vi "Read BMP File Data (excel).vi"(8 "error in (no error)":errorcluster, 11 "path to BMP file":path) -> (0 "error out":errorcluster, 1 "bitmap info":T1, 2 "color table":u32[](array[colorbox]), 3 "BMP data":u8[](array[numeric]))   [LabVIEW 2010, in "NI_ReportGenerationToolkit.lvlib"]
doc: "This VI reads in a Windows BMP file leaving the data packed as it was in the file. If no path is specified, a file dialog is used to find the file."
uses:
  <vilib>/addons/_office/NI_ReportGenerationToolkit.lvlib
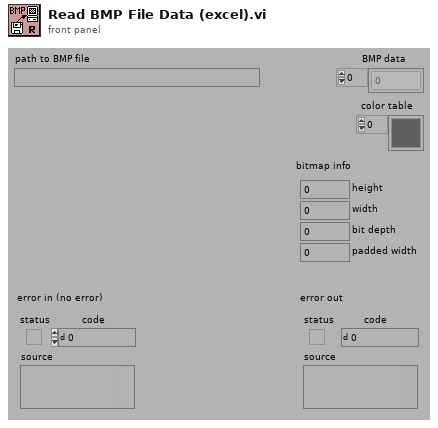
[diagram p1: front panel]
types:
  T1 = cluster{"height":u32, "width":u32, "bit depth":u16, "padded width":u32}
  T2 = enum16{"read/write", "read-only", "write-only", "write-only (truncate)"}
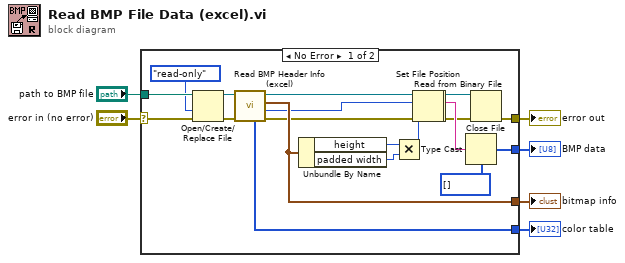
[diagram p0: block diagram]
diagram:
  n1 = case shown="No Error" "error in (no error)" {
    selector: "error in (no error)" -> [w9 w28]
    tunnel: "path to BMP file" -> [w26 _]
    tunnel: [w24 _] -> w5
    tunnel: [w22 _] -> w4
    tunnel: [w14 _] -> w3
    tunnel: [w11 w28] -> w2
    frame No Error {
      n2 = Open/Create/Replace File(file path (use dialog)=w26, error in=w9, access (0:read/write)=T2."read-only" ("open mode (0)")) -> (refnum out=w27:refnum<file>, error out=w19:errorcluster)  [unwired: 4 out]
      n3 = call <vilib>:"Read BMP Header Info (excel).vi"("error in (no error)"=w19, "BMP file"=w27) -> ("error out"=w13:errorcluster, "offset to data"=w23:u32, "bitmap info"=w24:T1, "BMP file"=w25:refnum<file>, "color table"=w22:u32[])  [unwired: 5 out]
      n4 = Unbundle By Name(w24) -> ("height"=w15:u32, "padded width"=w18:u32)
      n5 = Multiply(x=w15, y=w18) -> (x*y=w17:u32)
      n6 = Set File Position(offset (in bytes) (0)=w23, refnum=w25, error in=w13) -> (refnum out=w8:refnum<file>, error out=w7:errorcluster)  [unwired: 1 out]
      n7 = Read from Binary File(8:w7, 10:w17, 11:w8) -> (0:w12:errorcluster, 2:w16:string, 3:w21:refnum<file>)  [unwired: 4 out]
      n8 = Type Cast(type=u8[] [] ("array of bytes"), x=w16) -> (*(type *) &x=w14:u8[])
      n9 = Close File(refnum=w21, error in=w12) -> (error out=w11:errorcluster)  [unwired: 1 out]
    }
    frame Error {
    }
  }
  "error out" <- w2
  "bitmap info" <- w5
  "color table" <- w4
  "BMP data" <- w3
